vi "OSSCAR_stop_global_BM.vi"() -> ()   [LabVIEW 2021]
panel:
  out "OSSCAR_stop":bool
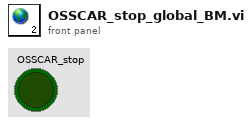
[diagram p1: front panel]
diagram:
